vi "TestVariables.vi"() -> ()   [LabVIEW 2020]
uses:
  D:/JemsTS_8.40.00/Module_Interfaces/ScriptVariableSpaceInterface.dll
  JemsTS_8.40.00/Module_Interfaces/ScriptVariableSpaceInterface.dll
panel:
  in  "reference":refnum<k24>
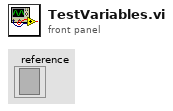
[diagram p1: front panel]
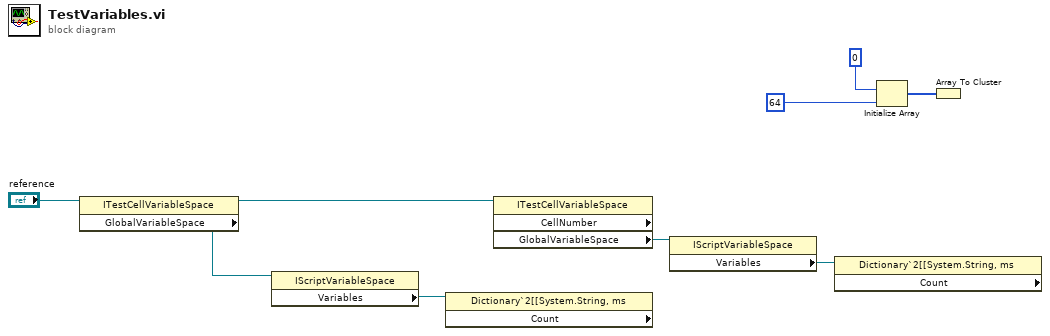
[diagram p0: block diagram]
diagram:
  n1 = property class="ITestCellVariableSpace"(reference="reference") -> (reference out=w6:refnum<k24>, "GlobalVariableSpace"=w8:refnum<k24>)  [unwired: 1 in, 1 out]
  n2 = property class="IScriptVariableSpace"(reference=w8) -> ("Variables"=w7:refnum<k24>)  [unwired: 1 in, 2 out]
  n3 = property class="Dictionary`2[[System.String, ms" props=["Count"](reference=w7) -> ()  [unwired: 1 in, 3 out]
  n4 = property class="ITestCellVariableSpace" props=["CellNumber", "GlobalVariableSpace"](reference=w6) -> ("GlobalVariableSpace"=w5:refnum<k24>)  [unwired: 1 in, 3 out]
  n5 = property class="IScriptVariableSpace"(reference=w5) -> ("Variables"=w4:refnum<k24>)  [unwired: 1 in, 2 out]
  n6 = property class="Dictionary`2[[System.String, ms" props=["Count"](reference=w4) -> ()  [unwired: 1 in, 3 out]
  n7 = Initialize Array(u8 0 ("new element/subarray"), 64 ("dimension size")) -> (w3:u8[])
  n8 = Array To Cluster(array=w3) -> ()  [unwired: 1 out]
